vi "QuickSearch Engine.vi"(0 "Owning Application":refnum<vi>, 1 "Exit Command":refnum<user-event>, 2 "Selected String":refnum<user-event>, 3 "New Match List":refnum<user-event>, 5 "Owning VI":refnum<vi>, 7 "Object Name":refnum<vi>, 9 "Name Match List":refnum<vi>) -> ()   [LabVIEW 2018]
uses:
  <vilib>/event_ctls.llb/eventvkey.ctl
panel:
  out "Shortcuts":string[](array[string])
  out "Name":string
  in  "Done":bool
  # "diagrama"
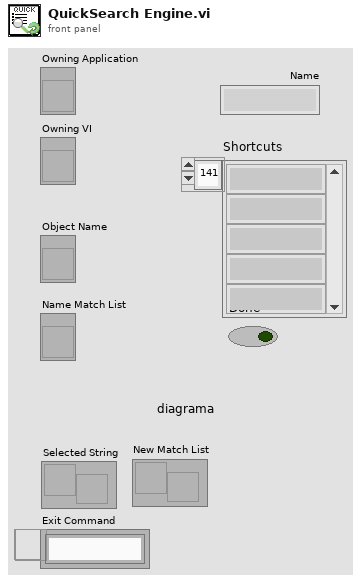
[diagram p1: front panel]
types:
  T1 = cluster{"OwningApp":refnum<event-registration>, "OwningVI":refnum<event-registration>, "Name Entry":refnum<event-registration>, "List":refnum<event-registration>, "List Pane":refnum<event-registration>, "User":refnum<event-registration>, "FOO":refnum<event-registration>}
  T2 = typedef "eventvkey.ctl" = enum16{"ASCII", "Enter", "Return", "Shift", "Ctrl", "Alt", "Cmd", "Opt", "Caps", "NumLock", "Clear", "Break", "Up", "Down", "Left", "Right", "Insert", "Delete", "Home", "End", "PageUp", "PageDown", "Escape", "Help", "Pause", "ScrollLock", "F1", "F2", "F3", "F4", "F5", "F6", "F7", "F8", "F9", "F10", "F11", "F12", "F13", "F14", "F15", "F16", "F17", "F18", "F19", "F20", "F21", "F22", "F23", "F24", "Play", "VolumeUp", "VolumeDown", "Mute", "Two Byte Char"}
  T3 = typedef "LVPoint32TypeDef.ctl" = cluster{"Horizontal":i32, "Vertical":i32}
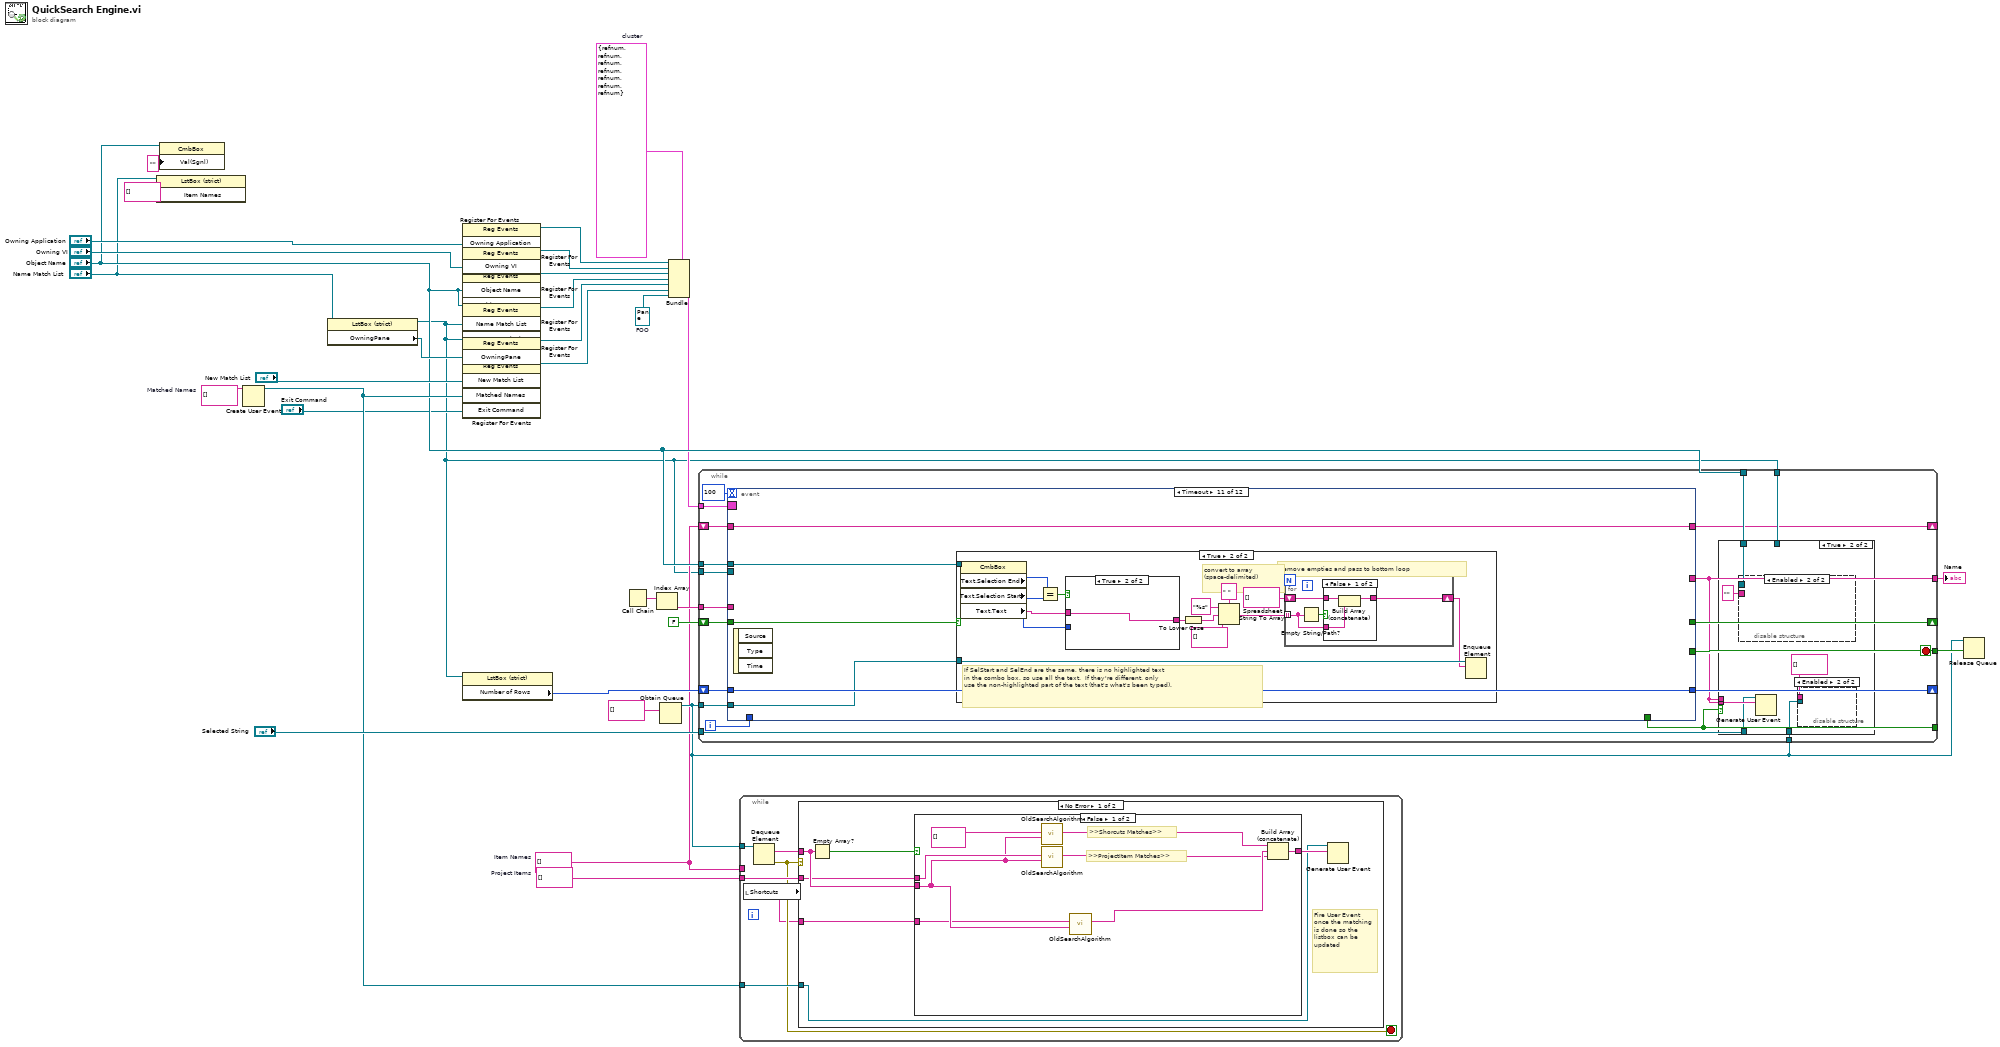
[diagram p0: block diagram]
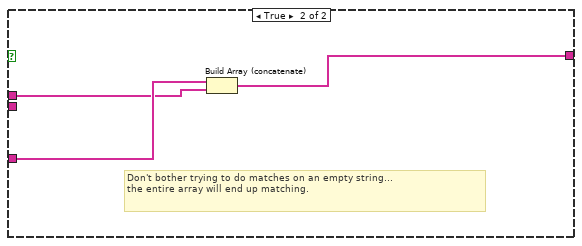
[diagram p2: hidden frame]
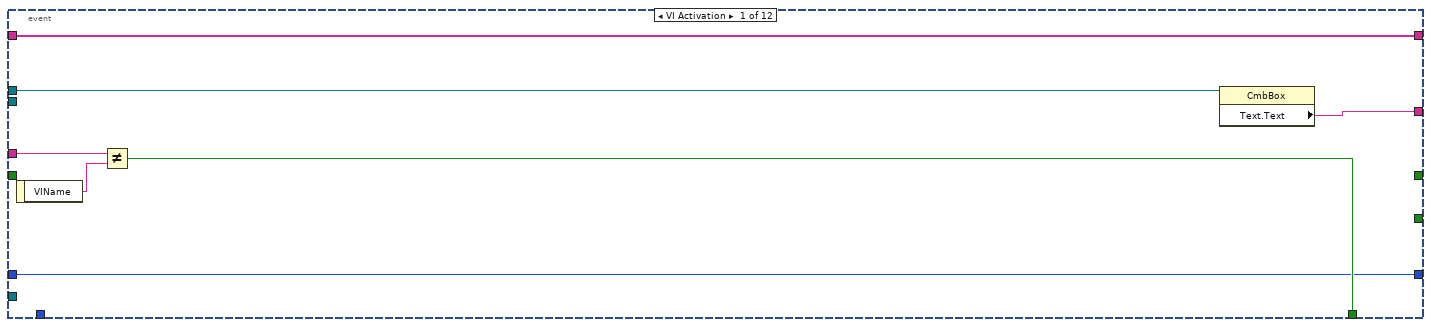
[diagram p4: hidden frame]
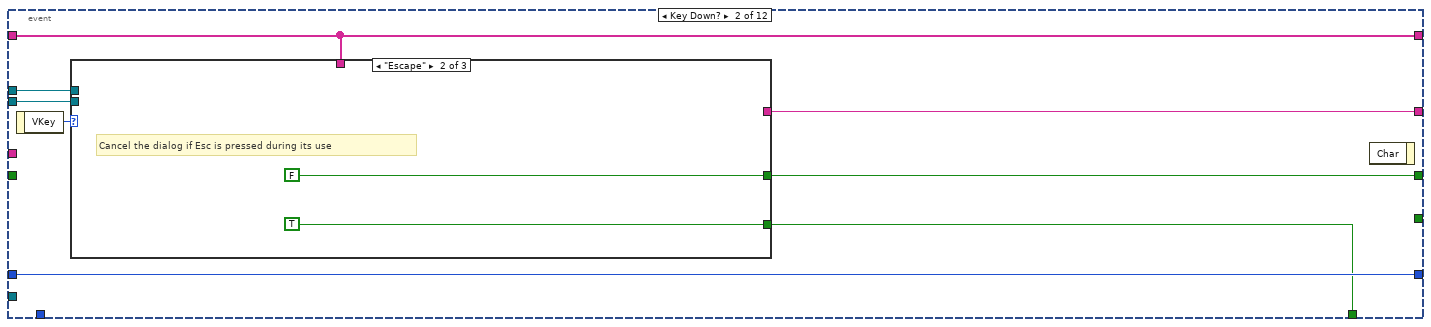
[diagram p5: hidden frame]
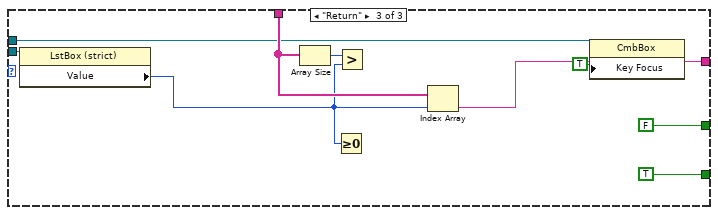
[diagram p7: hidden frame]
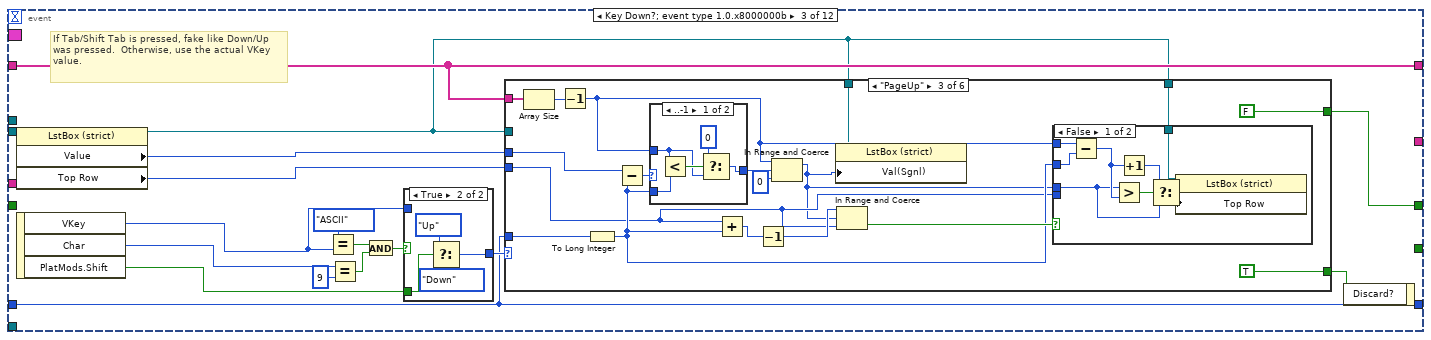
[diagram p8: hidden frame]
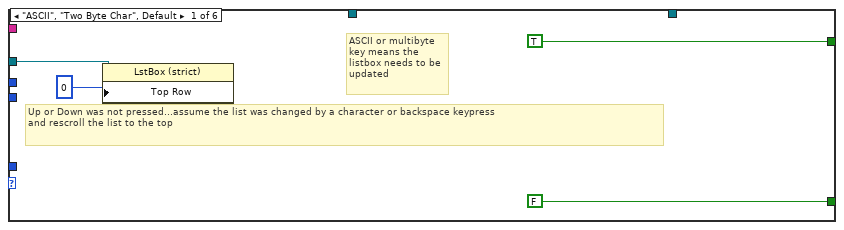
[diagram p10: hidden frame]
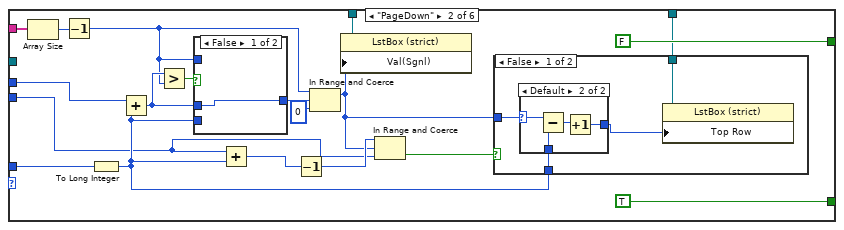
[diagram p11: hidden frame]
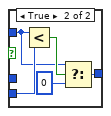
[diagram p12: hidden frame]
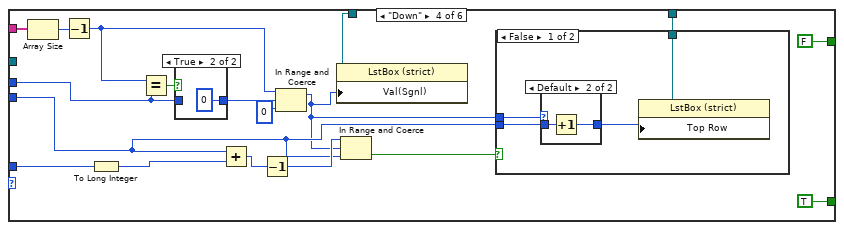
[diagram p17: hidden frame]
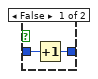
[diagram p18: hidden frame]
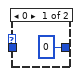
[diagram p19: hidden frame]
diagram:
  w1 = T1 {"OwningApp"=refnum, "OwningVI"=refnum, "Name Entry"=refnum, "List"=refnum, "List Pane"=refnum, "User"=refnum, "FOO"=refnum}  # cluster
  w2 = refnum<event-registration> refnum  # FOO
  w6 = string[] []  # Item Names
  w30 = string[] []  # Project Items
  w4 = string[] []  # Matched Names
  n1 = property class="LstBox (strict)"(reference="Name Match List", "Item Names"=string[] []) -> ()  [unwired: 1 in, 2 out]
  n2 = property class="CmbBox"(reference="Object Name", "Val(Sgnl)"="" ("Value (Signaling)")) -> ()  [unwired: 1 in, 2 out]
  n3 = Create User Event(user event datatype=w4) -> (user event=w17:refnum<user-event>)  [unwired: 1 in, 1 out]
  n4 = property class="LstBox (strict)"(reference="Name Match List") -> (reference out=w5:refnum<vi>, "OwningPane"=w19:refnum<vi>)  [unwired: 1 in, 1 out]
  n5 = register-events("Owning Application") -> (reference out=w14:refnum<event-registration>)  [unwired: 2 in, 1 out]
  n6 = register-events("Owning VI") -> (reference out=w13:refnum<event-registration>)  [unwired: 2 in, 1 out]
  n7 = register-events("Object Name", "Object Name") -> (reference out=w12:refnum<event-registration>)  [unwired: 2 in, 1 out]
  n8 = register-events(w5, w5) -> (reference out=w11:refnum<event-registration>)  [unwired: 2 in, 1 out]
  n9 = register-events(w19) -> (reference out=w10:refnum<event-registration>)  [unwired: 2 in, 1 out]
  n10 = register-events("New Match List", w17, "Exit Command") -> (reference out=w9:refnum<event-registration>)  [unwired: 2 in, 1 out]
  n11 = property on="Property Node" class="LstBox (strict)"(reference=w5) -> ("Number of Rows"=w27:u32)  [unwired: 1 in, 2 out]
  n12 = Call Chain() -> (call chain=w25:string[])
  n13 = Index Array(array=w25) -> (element=w26:string)  [unwired: 1 in]
  n14 = Obtain Queue(element data type=string[] []) -> (queue out=w22:refnum<queue>)  [unwired: 4 in, 2 out]
  n15 = Bundle(cluster=w1, "OwningApp"=w14, "OwningVI"=w13, "Name Entry"=w12, "List"=w11, "List Pane"=w10, "User"=w9, "FOO"=w2) -> (w8:T1)
  n16 = while {
    tunnel: "Object Name" -> [w52]
    tunnel: [w38] -> w24
    tunnel: w8 -> [w51]
    shift-right: [w35] -> _
    shift-left: w6 -> [w50]
    tunnel: w26 -> [w49]
    shift-right: [w47] -> _
    shift-left: w27 -> [w48]
    tunnel: w22 -> [w45]
    shift-right: [w43] -> _
    shift-left: FALSE -> [w44]
    tunnel: w5 -> [w42]
    tunnel: [w39] -> _
    tunnel: [w41] -> w31
    tunnel: "Selected String" -> [w40]
    tunnel: "Object Name" -> [w37]
    tunnel: w5 -> [w36]
    tunnel: w22 -> [w34]
    i -> [w33]
    stop <- w41 stop-if-true
    n17 = event shown="[10] Timeout" {
      selector: w51 -> [_ _ _ _ _ _ _ _ _ _ _ _]
      dyn-events: _ -> [_ _ _ _ _ _ _ _ _ _ _ _]
      timeout: 100 -> [_ _ _ _ _ _ _ _ _ _ _ _]
      tunnel: [w54 w64 _ w233 _ _ _ _ _ TRUE ("Discard?") _ w312] -> w39
      tunnel: w52 -> [w56 w60 _ _ w249 w255 _ _ _ w277 w279 _]
      tunnel: [w55 w61 _ w232 _ _ _ _ _ w276 _ _] -> w38
      tunnel: w50 -> [w59 w63 w83 w234 w248 w257 w261 _ _ w274 w282 w311]
      tunnel: [w59 w63 w83 w234 w248 w257 w261 w265 w268 w274 w282 w311] -> w35
      tunnel: w49 -> [w58 _ _ _ _ _ _ _ _ _ _ _]
      tunnel: w48 -> [w53 w67 w80 w231 w246 _ w260 w267 w270 w273 w281 w310]
      tunnel: [w53 w67 w80 w231 w246 w254 w260 w267 w270 w273 w281 w310] -> w47
      tunnel: w45 -> [_ _ _ _ _ _ _ _ _ _ w280 _]
      tunnel: w44 -> [_ _ _ _ _ w253 _ w264 w271 _ w278 _]
      tunnel: [_ w65 w82 _ FALSE w253 FALSE w264 w271 FALSE ("Discard?") _ TRUE] -> w43
      tunnel: w42 -> [_ w62 w95 _ _ w252 _ w266 w269 _ _ _]
      tunnel: [_ _ _ _ _ _ TRUE _ _ _ _ _] -> w41
      tunnel: w33 -> [_ _ _ _ _ _ _ _ _ _ _ _]
      event VI Activation {
        n18 = event-data() -> ("VIName"=w57:string)  [unwired: 1 in]
        n19 = Not Equal?(x=w58, y=w57) -> (x != y?=w54:bool)
        n20 = property on="Property Node" class="CmbBox"(reference=w56) -> ("Text.Text"=w55:string)  [unwired: 1 in, 2 out]
      }
      event Key Down? {
        n21 = event-data() -> ("VKey"=w66:T2)  [unwired: 1 in]
        n22 = case shown="\"Escape\"" w66 {
          tunnel: [_ FALSE FALSE] -> w65
          tunnel: [_ TRUE TRUE] -> w64
          tunnel: w63 -> [_ _ w75]
          tunnel: w62 -> [_ _ w74]
          tunnel: [_ _ w72] -> w61
          tunnel: w60 -> [_ _ w71]
          frame Default {
          }
          frame "Escape" {
            # "Cancel the dialog if Esc is pressed during its use"
          }
          frame "Return" {
            n23 = property class="LstBox (strict)"(reference=w74) -> ("Value"=w73:i32)  [unwired: 1 in, 2 out]
            n24 = Array Size(array=w75) -> (size(s)=w76:i32)
            n25 = Greater Or Equal To 0?(x=w73) -> ()  [unwired: 1 out]
            n26 = Greater?(x=w76, y=w73) -> ()  [unwired: 1 out]
            n27 = Index Array(array=w75, index=w73) -> (element=w72:string)
            n28 = property class="CmbBox"(reference=w71, "Key Focus"=TRUE) -> ()  [unwired: 1 in, 2 out]
          }
        }
        n29 = event-data() -> ()  [unwired: 2 in, 1 out]
      }
      event Key Down?; event type 1.0.x8000000b {
        # "If Tab/Shift Tab is pressed, fake like Down/Up was pressed.  Otherwise, use the actual VKey value."
        n30 = property on="Property Node" class="LstBox (strict)"(reference=w95) -> (reference out=w79:refnum<vi>, "Value"=w85:i32, "Top Row"=w84:i32)  [unwired: 1 in, 1 out]
        n31 = event-data() -> ("VKey"=w88:T2, "Char"=w87:i16, "PlatMods.Shift"=w86:bool)  [unwired: 1 in]
        n32 = Equal?(x=eventvkey."ASCII", y=w88) -> (x = y?=w91:bool)
        n33 = Equal?(x=w87, y=i16 9 ("x")) -> (x = y?=w92:bool)
        n34 = And(x=w91, y=w92) -> (x .and. y?=w90:bool)
        n35 = case shown="True" w90 {
          tunnel: w88 -> [w96 _]
          tunnel: [w96 w97] -> w89
          tunnel: w86 -> [_ w100]
          frame False {
          }
          frame True {
            n36 = Select(t=eventvkey."Up" ("x"), s=w100, f=eventvkey."Down" ("x")) -> (s? t:f=w97:T2)
          }
        }
        n37 = case shown="\"PageUp\"" w89 {
          tunnel: w80 -> [_ w115 w147 w179 w207 _]
          tunnel: [FALSE TRUE TRUE TRUE TRUE w230] -> w81
          tunnel: w83 -> [_ w119 w151 w183 w211 _]
          tunnel: [TRUE FALSE FALSE FALSE FALSE w230] -> w82
          tunnel: w85 -> [_ w109 w143 w175 w203 _]
          tunnel: w84 -> [_ w108 w142 w174 w202 _]
          tunnel: w79 -> [_ w105 w139 w171 w199 _]
          tunnel: w79 -> [_ w107 w141 w172 w201 _]
          tunnel: w79 -> [w102 _ _ _ _ _]
          frame "ASCII", "Two Byte Char", Default {
            # "ASCII or multibyte key means the listbox needs to be updated"
            # "Up or Down was not pressed...assume the list was changed by a character or backspace keypress\nand rescroll the list to the top"
            n38 = property on="Property Node" class="LstBox (strict)"(reference=w102, "Top Row"=0) -> ()  [unwired: 1 in, 2 out]
          }
          frame "PageDown" {
            n39 = Array Size(array=w119) -> (size(s)=w118:i32)
            n40 = Decrement(x=w118) -> (x-1=w111:i32)
            n41 = To Long Integer(number=w115) -> (32bit integer=w110:i32)
            n42 = Add(x=w109, y=w110) -> (x+y=w113:i32)
            n43 = Greater?(x=w113, y=w111) -> (0:w114:bool)
            n44 = case shown="False" w114 {
              tunnel: w113 -> [w124 _]
              tunnel: [w124 w128] -> w112
              tunnel: w111 -> [_ w126]
              tunnel: w110 -> [_ w129]
              frame False {
              }
              frame True {
                n45 = Less?(x=w126, y=w129) -> (x < y?=w127:bool)
                n46 = Select(t=w126, s=w127, f=0 ("y")) -> (s? t:f=w128:i32)
              }
            }
            n47 = Add(x=w108, y=w110) -> (x+y=w123:i32)
            n48 = Decrement(x=w123) -> (x-1=w121:i32)
            n49 = In Range and Coerce(upper limit=w111, x=w112, lower limit=0 ("y")) -> (coerced(x)=w106:i32)  [unwired: 1 out]
            n50 = property on="Property Node" class="LstBox (strict)"(reference=w107, "Val(Sgnl)"=w106) -> ()  [unwired: 1 in, 2 out]
            n51 = In Range and Coerce(upper limit=w121, x=w106, lower limit=w108) -> (In Range?=w122:bool)  [unwired: 1 out]
            n52 = case shown="False" w122 {
              tunnel: w106 -> [w132 _]
              tunnel: w110 -> [w133 _]
              tunnel: w105 -> [w131 _]
              frame False {
                n53 = case shown="Default" w132 {
                  selector: w132 -> [w134 w135]
                  tunnel: [w134 w138] -> w130
                  tunnel: w133 -> [_ w137]
                  frame 0 {
                  }
                  frame Default {
                    n54 = Subtract(x=w135, y=w137) -> (x-y=w136:i32)
                    n55 = Increment(x=w136) -> (x+1=w138:i32)
                  }
                }
                n56 = property on="Property Node" class="LstBox (strict)"(reference=w131, "Top Row"=w130) -> ()  [unwired: 1 in, 2 out]
              }
              frame True {
                # "The newly selected item is visible, so no scrolling is necessary"
              }
            }
          }
          frame "PageUp" {
            n57 = Array Size(array=w151) -> (size(s)=w150:i32)
            n58 = Decrement(x=w150) -> (x-1=w146:i32)
            n59 = To Long Integer(number=w147) -> (32bit integer=w144:i32)
            n60 = Subtract(x=w143, y=w144) -> (x-y=w145:i32)
            n61 = case shown="..-1" w145 {
              selector: w145 -> [_ w162]
              tunnel: [w158 w162] -> w153
              tunnel: w146 -> [w159 _]
              tunnel: w144 -> [w161 _]
              frame ..-1 {
                n62 = Less?(x=w159, y=w161) -> (x < y?=w160:bool)
                n63 = Select(t=0, s=w160, f=w159) -> (s? t:f=w158:i32)
              }
              frame 0.. {
              }
            }
            n64 = Add(x=w142, y=w144) -> (x+y=w156:i32)
            n65 = Decrement(x=w156) -> (x-1=w154:i32)
            n66 = In Range and Coerce(upper limit=w146, x=w153, lower limit=0 ("y")) -> (coerced(x)=w140:i32)  [unwired: 1 out]
            n67 = property on="Property Node" class="LstBox (strict)"(reference=w141, "Val(Sgnl)"=w140) -> ()  [unwired: 1 in, 2 out]
            n68 = In Range and Coerce(upper limit=w154, x=w140, lower limit=w142) -> (In Range?=w155:bool)  [unwired: 1 out]
            n69 = case shown="False" w155 {
              tunnel: w142 -> [_ _]
              tunnel: w140 -> [w166 _]
              tunnel: w146 -> [w170 _]
              tunnel: w144 -> [w169 _]
              tunnel: w139 -> [w164 _]
              frame False {
                n70 = Subtract(x=w170, y=w169) -> (x-y=w167:i32)
                n71 = Greater?(x=w166, y=w167) -> (0:w168:bool)
                n72 = Increment(x=w167) -> (x+1=w165:i32)
                n73 = Select(t=w165, s=w168, f=w166) -> (s? t:f=w163:i32)
                n74 = property on="Property Node" class="LstBox (strict)"(reference=w164, "Top Row"=w163) -> ()  [unwired: 1 in, 2 out]
              }
              frame True {
                # "The newly selected item is visible, so no scrolling is necessary"
              }
            }
          }
          frame "Down" {
            n75 = Array Size(array=w183) -> (size(s)=w182:i32)
            n76 = Decrement(x=w182) -> (x-1=w177:i32)
            n77 = To Long Integer(number=w179) -> (32bit integer=w178:i32)
            n78 = Equal?(x=w177, y=w175) -> (x = y?=w176:bool)
            n79 = case shown="True" w176 {
              tunnel: [w190 0] -> w185
              tunnel: w175 -> [w189 _]
              frame False {
                n80 = Increment(x=w189) -> (x+1=w190:i32)
              }
              frame True {
              }
            }
            n81 = Add(x=w174, y=w178) -> (x+y=w188:i32)
            n82 = Decrement(x=w188) -> (x-1=w186:i32)
            n83 = In Range and Coerce(upper limit=w177, x=w185, lower limit=0 ("y")) -> (coerced(x)=w173:i32)  [unwired: 1 out]
            n84 = property on="Property Node" class="LstBox (strict)"(reference=w172, "Val(Sgnl)"=w173) -> ()  [unwired: 1 in, 2 out]
            n85 = In Range and Coerce(upper limit=w186, x=w173, lower limit=w174) -> (In Range?=w187:bool)  [unwired: 1 out]
            n86 = case shown="False" w187 {
              tunnel: w174 -> [w195 _]
              tunnel: w173 -> [w194 _]
              tunnel: w171 -> [w192 _]
              frame False {
                n87 = case shown="Default" w194 {
                  tunnel: w195 -> [_ w198]
                  tunnel: [0 w197] -> w193
                  frame 0 {
                  }
                  frame Default {
                    n88 = Increment(x=w198) -> (x+1=w197:i32)
                  }
                }
                n89 = property on="Property Node" class="LstBox (strict)"(reference=w192, "Top Row"=w193) -> ()  [unwired: 1 in, 2 out]
              }
              frame True {
                # "The newly selected item is visible, so no scrolling is necessary"
              }
            }
          }
          frame "Up" {
            n90 = Array Size(array=w211) -> (size(s)=w210:i32)
            n91 = Decrement(x=w210) -> (x-1=w205:i32)
            n92 = To Long Integer(number=w207) -> (32bit integer=w206:i32)
            n93 = Decrement(x=w203) -> (x-1=w204:i32)
            n94 = case shown="..-1" w204 {
              selector: w204 -> [_ w218]
              tunnel: [w217 w218] -> w213
              tunnel: w205 -> [w217 _]
              frame ..-1 {
              }
              frame 0.. {
              }
            }
            n95 = Add(x=w202, y=w206) -> (x+y=w216:i32)
            n96 = Decrement(x=w216) -> (x-1=w214:i32)
            n97 = In Range and Coerce(upper limit=w205, x=w213, lower limit=0 ("y")) -> (coerced(x)=w200:i32)  [unwired: 1 out]
            n98 = In Range and Coerce(upper limit=w214, x=w200, lower limit=w202) -> (In Range?=w215:bool)  [unwired: 1 out]
            n99 = property on="Property Node" class="LstBox (strict)"(reference=w201, "Val(Sgnl)"=w200) -> ()  [unwired: 1 in, 2 out]
            n100 = case shown="False" w215 {
              tunnel: w202 -> [w223 _]
              tunnel: w206 -> [w222 _]
              tunnel: w205 -> [w221 _]
              tunnel: w199 -> [w219 _]
              frame False {
                n101 = case shown="..0" w223 {
                  selector: w223 -> [_ w228]
                  tunnel: [w224 w229] -> w220
                  tunnel: w222 -> [w226 _]
                  tunnel: w221 -> [w227 _]
                  frame ..0 {
                    n102 = Subtract(x=w227, y=w226) -> (x-y=w225:i32)
                    n103 = Increment(x=w225) -> (x+1=w224:i32)
                  }
                  frame 1.. {
                    n104 = Decrement(x=w228) -> (x-1=w229:i32)
                  }
                }
                n105 = property on="Property Node" class="LstBox (strict)"(reference=w219, "Top Row"=w220) -> ()  [unwired: 1 in, 2 out]
              }
              frame True {
                # "The newly selected item is visible, so no scrolling is necessary"
              }
            }
          }
          frame "Shift" {
            w230 = FALSE
            # "Shift should not trigger the bottom loop to do a search."
          }
        }
        n106 = event-data("Discard?"=w81) -> ()  [unwired: 1 in, 1 out]
      }
      event Mouse Up {
        # "Conditions:\n1.  Mouse Up was not in empty space after the last row.\n2.  Mouse Up was not on scrollbars.\n3.  A valid row is selected in the listbox.\n4.  This was the second Mouse Up from a double click."
        n107 = event-data() -> ("CtlRef"=w235:refnum<vi>, "Coords"=w236:T3, "Mods.Double Click"=w237:bool)  [unwired: 1 in]
        n108 = invoke on="Invoke Node" class="LstBox (strict)" method="Point To Row"(reference=w235, "Point"=w236) -> ("InBounds"=w238:bool, "Row"=w242:i32)  [unwired: 5 in, 5 out]
        n109 = Array Size(array=w234) -> (size(s)=w240:i32)
        n110 = Greater Or Equal To 0?(x=w242) -> (x >= 0?=w239:bool)
        n111 = Greater?(x=w240, y=w242) -> (0:w241:bool)
        n112 = Compound Arithmetic op=AND(w241, w238, w239, w237) -> (w233:bool)
        n113 = Index Array(array=w234, index=w242) -> (element=w232:string)
      }
      event Value Change {
        # "A new value in the listbox should be reflected\nin the combo box.  This code sets the text\nin the combo box, highlights it, and sets\nkey focus."
        n114 = event-data() -> ("NewVal"=w247:i32)  [unwired: 1 in]
        n115 = Index Array(array=w248, index=w247) -> (element=w251:string)
        n116 = String Length(string=w251) -> (length=w250:i32)
        n117 = property on="Property Node" class="CmbBox"(reference=w249, "Text.Text"=w251, "Key Focus"=TRUE, "Text.Selection Start"=u32 0 ("Text.Selection:Start"), "Text.Selection End"=w250) -> ()  [unwired: 1 in, 2 out]
      }
      event Pane Size {
        n118 = event-data() -> ()  [unwired: 1 in, 1 out]
        n119 = property on="Property Node" class="CmbBox" props=["Width"](reference=w255) -> (error out=w256:errorcluster)  [unwired: 1 in, 2 out]
        n120 = property on="Property Node" class="LstBox (strict)"(reference=w252, error in=w256) -> ("Number of Rows"=w254:u32)  [unwired: 2 out]
      }
      event User Event {
        n121 = event-data() -> ()  [unwired: 1 in, 1 out]
      }
      event User Event {
        # "The name matching is done...update the listbox with the new matched names"
        n122 = event-data() -> ("Matched Names"=w265:string[])  [unwired: 1 in]
        n123 = property on="Property Node" class="LstBox (strict)"(reference=w266, "Item Names"=w265) -> (reference out=w263:refnum<vi>)  [unwired: 1 in, 1 out]
        n124 = property class="LstBox (strict)"(reference=w263, "Value"=-1 ("Name Match List")) -> ()  [unwired: 1 in, 2 out]
      }
      event User Event {
        n125 = event-data() -> ("All NV Strings"=w268:string[])  [unwired: 1 in]
        "Shortcuts" <- w268
        n126 = property class="LstBox (strict)"(reference=w269, "Item Names"=w268) -> ()  [unwired: 1 in, 2 out]
      }
      event "Done": Value Change {
        # "The Done button is off-screen, but has Enter set for Key Focus.  So if Enter is pressed, it acts like a commit."
        n127 = event-data() -> ()  [unwired: 1 in, 2 out]
        n128 = property on="Property Node" class="CmbBox"(reference=w277) -> ("Text.Text"=w276:string)  [unwired: 1 in, 2 out]
      }
      event Timeout {
        n129 = event-data() -> ()  [unwired: 1 in, 3 out]
        n130 = case shown="True" w278 {
          tunnel: w280 -> [_ w296]
          tunnel: w279 -> [_ w283]
          frame False {
            # "No need to update the listbox"
          }
          frame True {
            # "Remove empties and pass to bottom loop"
            # "convert to array\n(space-delimited)"
            # "If SelStart and SelEnd are the same, there is no highlighted text\nin the combo box, so use all the text.  If they're different, only\nuse the non-highlighted part of the text (that's what's been typed)."
            n131 = property on="Property Node" class="CmbBox"(reference=w283) -> ("Text.Selection End"=w295:u32, "Text.Selection Start"=w292:u32, "Text.Text"=w291:string)  [unwired: 1 in, 2 out]
            n132 = Equal?(x=w295, y=w292) -> (x = y?=w294:bool)
            n133 = case shown="True" w294 {
              tunnel: [w307 w308] -> w293
              tunnel: w292 -> [w306 _]
              tunnel: w291 -> [w305 w308]
              frame False {
                n134 = String Subset(string=w305, length (rest)=w306) -> (substring=w307:string)  [unwired: 1 out]
              }
              frame True {
              }
            }
            n135 = To Lower Case(string=w293) -> (all lower case string=w288:string)
            n136 = Spreadsheet String To Array(delimiter (Tab)=" ", format string="%s", spreadsheet string=w288, array type (2D Dbl)=string[] []) -> (array=w286:string[])
            n137 = for {
              tunnel: w286 -> [w297] mode=indexing
              shift-right: [w298] -> w284
              shift-left: string[] [] -> [w299]
              n138 = Empty String/Path?(string/path=w297) -> (empty?=w300:bool)
              n139 = case shown="False" w300 {
                tunnel: w299 -> [w303 w304]
                tunnel: [w301 w304] -> w298
                tunnel: w297 -> [w302 _]
                frame False {
                  n140 = Build Array (concatenate)(w303, w302) -> (w301:string[])
                }
                frame True {
                }
              }
            }
            n141 = Enqueue Element(queue=w296, element=w284) -> ()  [unwired: 1 in, 4 out]
          }
        }
      }
      event Panel Close? {
        w312 = TRUE ("Discard?")
        n142 = event-data() -> ()  [unwired: 1 in, 1 out]
        n143 = event-data("Discard?"=w312) -> ()  [unwired: 1 in, 1 out]
      }
    }
    n144 = case shown="True" w39 {
      tunnel: w38 -> [_ w318]
      tunnel: w40 -> [_ w317]
      tunnel: w38 -> [_ _]
      tunnel: w37 -> [_ w315]
      tunnel: w36 -> [_ _]
      tunnel: w34 -> [_ w314]
      frame False {
      }
      frame True {
        n145 = disable-structure shown="Enabled" {
          disable-tunnel: "" ("Value (Signaling)") -> [w322 _]
          disable-tunnel: w315 -> [w321 _]
          frame Disabled {
            n146 = property class="CmbBox"(reference=w321, "Val(Sgnl)"=w322) -> ()  [unwired: 1 in, 2 out]
          }
          frame Enabled {
          }
        }
        n147 = Generate User Event(user event=w317, event data cluster=w318) -> ()  [unwired: 2 in, 2 out]
        n148 = disable-structure shown="Enabled" {
          disable-tunnel: w314 -> [w320 _]
          disable-tunnel: string[] [] ("element") -> [w319 _]
          frame Disabled {
            n149 = Enqueue Element(queue=w320, element=w319) -> ()  [unwired: 2 in, 3 out]
          }
          frame Enabled {
          }
        }
      }
    }
  }
  "Name" <- w24
  n150 = while {
    tunnel: w22 -> [w328]
    tunnel: w30 -> [w326]
    tunnel: w6 -> [_]
    tunnel: w17 -> [w325]
    stop <- w324 stop-if-true
    n151 = local read "Shortcuts"() -> (w323:string[])
    n152 = Dequeue Element(queue=w328) -> (element=w327:string[], error out=w324:errorcluster)  [unwired: 1 in, 3 out]
    n153 = case shown="No Error" w324 {
      tunnel: w327 -> [w333 _]
      tunnel: w326 -> [w332 _]
      tunnel: w323 -> [w331 _]
      tunnel: w325 -> [w329 _]
      frame No Error {
        # "Fire User Event once the matching is done so the listbox can be updated"
        n154 = Empty Array?(array=w333) -> (empty?=w334:bool)
        n155 = case shown="False" w334 {
          tunnel: w333 -> [w341 _]
          tunnel: [w337 w344] -> w330
          tunnel: w332 -> [w342 w343]
          tunnel: w331 -> [w336 w345]
          frame False {
            # ">>ProjectItem Matches>>"
            # ">>Shorcuts Matches>>"
            n156 = call <resource>:"OldSearchAlgorithm.vi"("Query terms"=w341, "SearchList Case"=string[] [] ("Shortcuts")) -> ("Search Result"=w339:string[])  [unwired: 9 in]
            n157 = call <resource>:"OldSearchAlgorithm.vi"("Query terms"=w341, "SearchList Case"=w342) -> ("Search Result"=w338:string[])  [unwired: 9 in]
            n158 = call <resource>:"OldSearchAlgorithm.vi"("Query terms"=w341, "SearchList Case"=w336) -> ("Search Result"=w340:string[])  [unwired: 9 in]
            n159 = Build Array (concatenate)(w339, w340, w338) -> (w337:string[])
          }
          frame True {
            # "Don't bother trying to do matches on an empty string...\nthe entire array will end up matching."
            n160 = Build Array (concatenate)(w345, w343) -> (w344:string[])
          }
        }
        n161 = Generate User Event(user event=w329, event data cluster=w330) -> ()  [unwired: 2 in, 2 out]
      }
      frame Error {
      }
    }
  }
  n162 = Release Queue(queue=w22, force destroy? (F)=w31) -> ()  [unwired: 1 in, 3 out]
